vi "Configure Dispense Time.vi"(8 "error in (no error)":errorcluster, 10 "Dispense Time (0000)":i32 format="%04.0f", 11 "VISA resource name":refnum<visa-resource-name>) -> (0 "error out":errorcluster, 3 "VISA resource name out":refnum<visa-resource-name>)   [LabVIEW 2020, in "EFD Ultimus V.lvlib"]
doc: "Updates the dispense time value in the current memory location. \n\nHost Format: PS--Tttttt\nttttt: The four or five digit dispense time value excluding the decimal point. The valid range is 0.0000 to 9.9999. This command accepts either 3 or 4 decimal places."
uses:
  EFD Ultimus V.lvlib
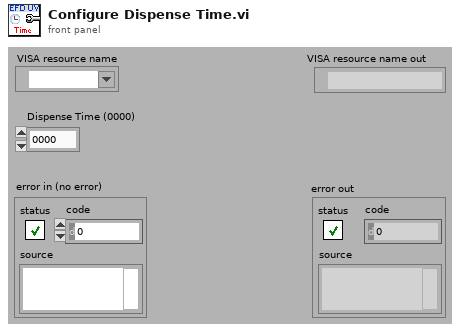
[diagram p1: front panel]
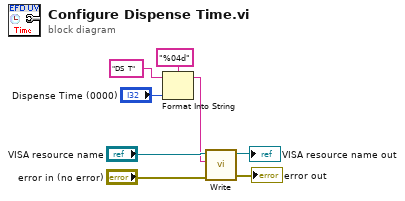
[diagram p0: block diagram]
diagram:
  n1 = Format Into String(format string="%04d", initial string="DS  T" ("string"), "Dispense Time (0000)") -> (resulting string=w3:string)  [unwired: 1 in, 1 out]
  n2 = call "Write.vi"("error in (no error)"="error in (no error)", "Command To Write"=w3, "VISA resource name"="VISA resource name") -> ("error out"=→"error out":errorcluster, "VISA resource name out"=→"VISA resource name out":refnum<visa-resource-name>)  [unwired: 7 out]
